vi "LDA_IP.vi"() -> (15 "error out":errorcluster)   [LabVIEW 2013]
uses:
  Globals/Meas_global.vi
  Globals/LDA_meas_global_1.vi
  Globals/LDA_meas_global_2.vi
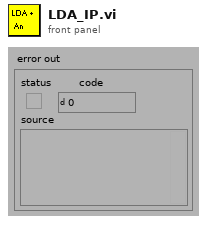
[diagram p1: front panel]
types:
  T1 = typedef "Ch_and_Spans.ctl" = cluster{"high limit (10V)":sgl, "low limit (-10V)":sgl, "Ch No":i16, "Var name":string, "Use Latest Calib":bool}
  T2 = typedef "LDA_Setup.ctl" = cluster{"dimensions":enum16{"1D", "2D"}, "Analogue Freq Multiplier":dbl}
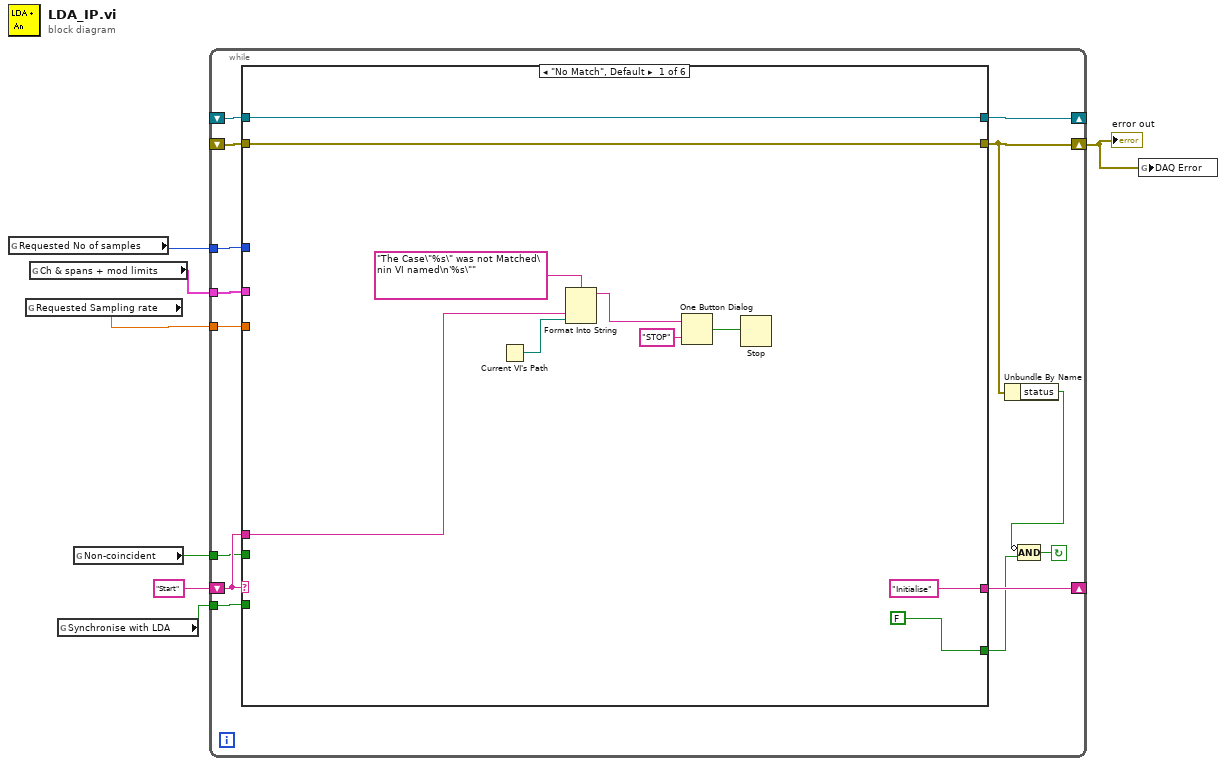
[diagram p0: block diagram]
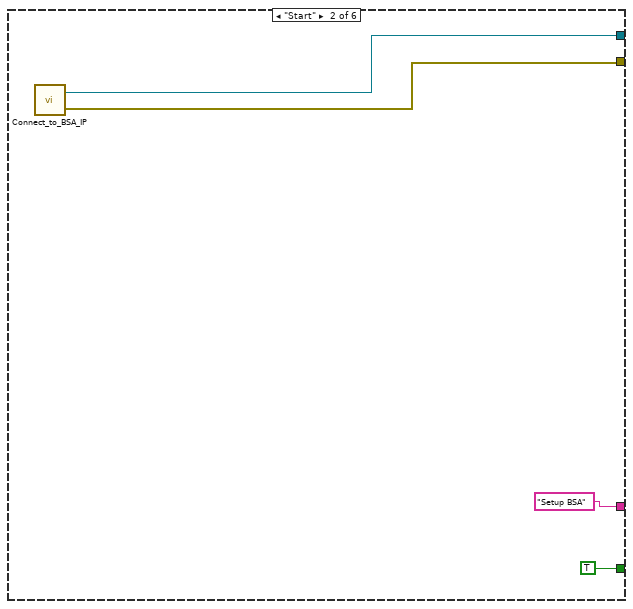
[diagram p2: hidden frame]
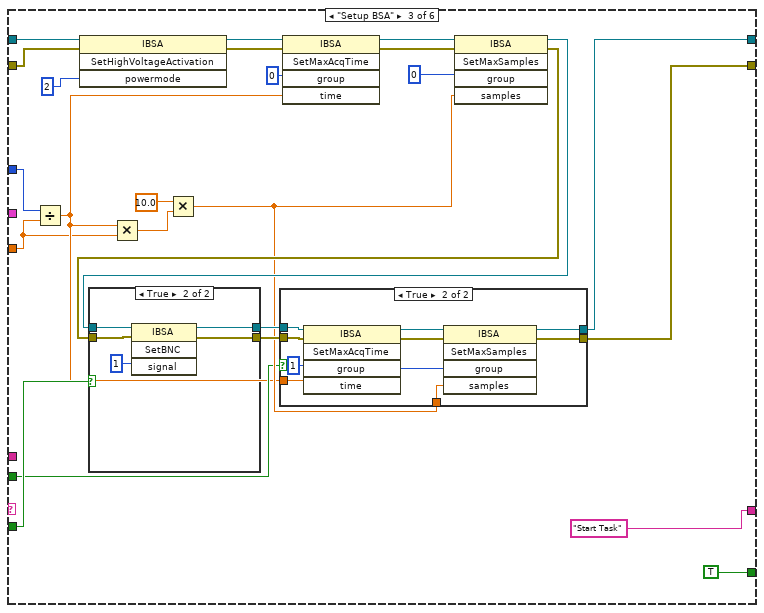
[diagram p3: hidden frame]
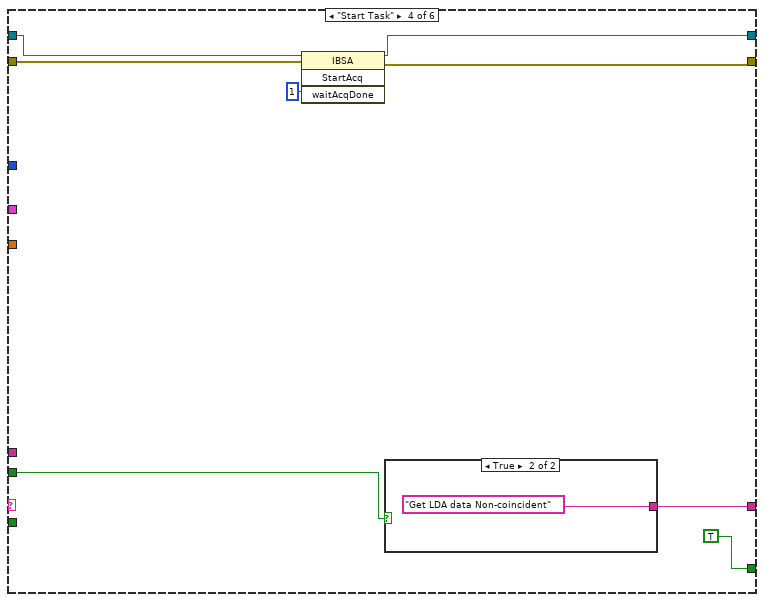
[diagram p6: hidden frame]
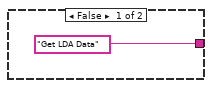
[diagram p7: hidden frame]
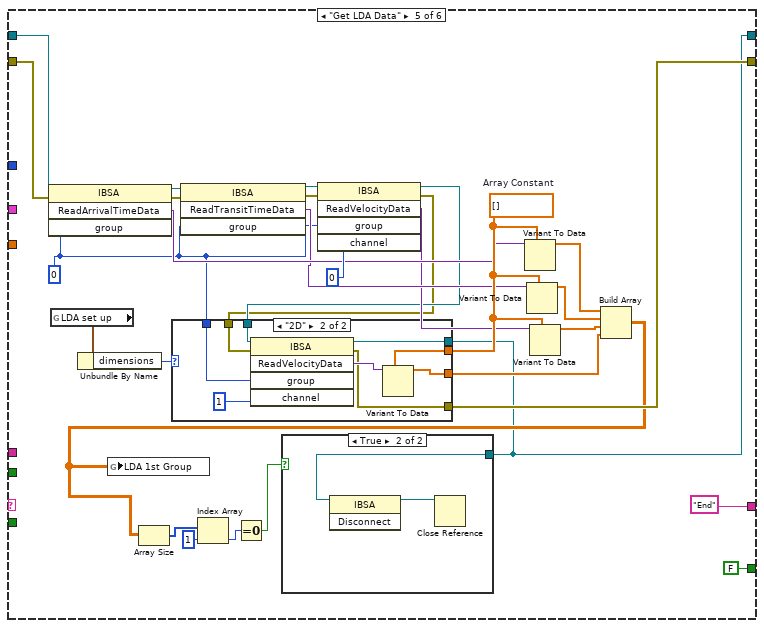
[diagram p8: hidden frame]
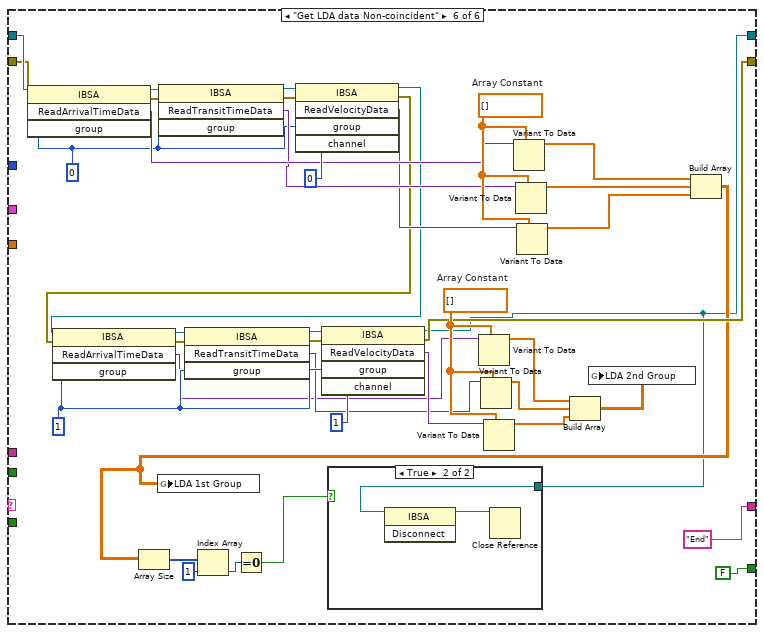
[diagram p11: hidden frame]
diagram:
  n1 = global read "Meas_global.vi" "Requested No of samples"() -> (w2:i32)
  n2 = global read "Meas_global.vi" "Requested Sampling rate"() -> (w3:dbl)
  n3 = global read "Meas_global.vi" "Ch & spans + mod limits"() -> (w4:T1[])
  n4 = global read "Meas_global.vi" "Synchronise with LDA"() -> (w6:bool)
  n5 = global read "LDA_meas_global_1.vi" "Non-coincident"() -> (w5:bool)
  n6 = while {
    shift-left: "Start" -> [w20]
    shift-right: [w21] -> _
    shift-right: [w11] -> w1
    shift-left: _ -> [w19]
    tunnel: w2 -> [w18]
    tunnel: w4 -> [w17]
    tunnel: w3 -> [w16]
    shift-right: [w14] -> _
    shift-left: _ -> [w15]
    tunnel: w6 -> [w13]
    tunnel: w5 -> [w12]
    stop <- w9 continue-if-true
    n7 = case shown="\"No Match\", Default" w20 {
      tunnel: [FALSE TRUE TRUE TRUE FALSE FALSE] -> w8
      tunnel: ["Initialise" "Setup BSA" "Start Task" w81 "End" "End"] -> w21
      tunnel: w20 -> [w26 _ _ _ _ _]
      tunnel: [w23 w33 w42 w85 w100 w142] -> w11
      tunnel: w19 -> [w23 _ w51 w82 w94 w140]
      tunnel: w18 -> [_ _ w52 _ _ _]
      tunnel: w17 -> [_ _ _ _ _ _]
      tunnel: w16 -> [_ _ w37 _ _ _]
      tunnel: w15 -> [w22 _ w53 w84 w104 w141]
      tunnel: [w22 w34 w44 w83 w90 w133] -> w14
      tunnel: w13 -> [_ _ w46 _ _ _]
      tunnel: w12 -> [_ _ w40 w80 _ _]
      frame "No Match", Default {
        n8 = Current VI's Path() -> (path=w25:path)
        n9 = Format Into String(format string="The Case\"%s\" was not Matched\nin VI named\n'%s\"" ("Format String"), w26, w25) -> (resulting string=w29:string)  [unwired: 2 in, 1 out]
        n10 = One Button Dialog(message=w29, button name ("OK")="STOP") -> (true=w27:bool)
        n11 = Stop(stop? (T)=w27) -> ()
      }
      frame "Start" {
        n12 = call "Connect_to_BSA_IP.vi"() -> ("error out"=w33:errorcluster, "BSA"=w34:refnum<k7>)  [unwired: 2 out]
      }
      frame "Setup BSA" {
        n13 = Divide(x=w52, y=w37) -> (x/y=w38:dbl)
        n14 = invoke class="IBSA" method="SetHighVoltageActivation"(reference=w53, error in=w51, "powermode"=2) -> (reference out=w58:refnum<k7>, error out=w60:errorcluster)  [unwired: 1 in, 2 out]
        n15 = Multiply(x=w38, y=w37) -> (x*y=w36:dbl)
        n16 = Multiply(x=10.0 ("y"), y=w36) -> (x*y=w41:dbl)
        n17 = invoke class="IBSA" method="SetMaxAcqTime"(reference=w58, error in=w60, "group"=0, "time"=w38) -> (reference out=w59:refnum<k7>, error out=w57:errorcluster)  [unwired: 1 in, 3 out]
        n18 = invoke class="IBSA" method="SetMaxSamples"(reference=w59, error in=w57, "group"=0, "samples"=w41) -> (reference out=w48:refnum<k7>, error out=w47:errorcluster)  [unwired: 1 in, 3 out]
        n19 = case shown="True" w46 {
          tunnel: w48 -> [w72 w77]
          tunnel: w47 -> [w73 w76]
          tunnel: [w72 w75] -> w45
          tunnel: [w73 w74] -> w43
          frame False {
          }
          frame True {
            n20 = invoke class="IBSA" method="SetBNC"(reference=w77, error in=w76, "signal"=1) -> (reference out=w75:refnum<k7>, error out=w74:errorcluster)  [unwired: 1 in, 2 out]
          }
        }
        n21 = case shown="True" w40 {
          tunnel: w45 -> [w62 w69]
          tunnel: [w62 w67] -> w44
          tunnel: w43 -> [w61 w66]
          tunnel: [w61 w65] -> w42
          tunnel: w38 -> [_ w64]
          tunnel: w41 -> [_ w63]
          frame False {
          }
          frame True {
            w70 = 1 ("group")
            n22 = invoke class="IBSA" method="SetMaxAcqTime"(reference=w69, error in=w66, "group"=w70, "time"=w64) -> (reference out=w68:refnum<k7>, error out=w71:errorcluster)  [unwired: 1 in, 3 out]
            n23 = invoke class="IBSA" method="SetMaxSamples"(reference=w68, error in=w71, "group"=w70, "samples"=w63) -> (reference out=w67:refnum<k7>, error out=w65:errorcluster)  [unwired: 1 in, 3 out]
          }
        }
      }
      frame "Start Task" {
        n24 = invoke class="IBSA" method="StartAcq"(reference=w84, error in=w82, "waitAcqDone"=1) -> (reference out=w83:refnum<k7>, error out=w85:errorcluster)  [unwired: 1 in, 2 out]
        n25 = case shown="True" w80 {
          tunnel: ["Get LDA Data" "Get LDA data Non-coincident"] -> w81
          frame False {
          }
          frame True {
          }
        }
      }
      frame "Get LDA Data" {
        w112 = dbl[] []  # Array Constant
        w101 = 0 ("group")
        n26 = invoke class="IBSA" method="ReadArrivalTimeData"(reference=w104, error in=w94, "group"=w101) -> (reference out=w117:refnum<k7>, error out=w116:errorcluster, "ReadArrivalTimeData"=w111:variant)  [unwired: 1 in, 1 out]
        n27 = global read "Meas_global.vi" "LDA set up"() -> (w93:T2)
        n28 = Unbundle By Name(w93) -> ("dimensions"=w92:enum16{"1D", "2D"})
        n29 = invoke class="IBSA" method="ReadTransitTimeData"(reference=w117, error in=w116, "group"=w101) -> (reference out=w115:refnum<k7>, error out=w114:errorcluster, "ReadTransitTimeData"=w110:variant)  [unwired: 1 in, 1 out]
        n30 = invoke class="IBSA" method="ReadVelocityData"(reference=w115, error in=w114, "group"=w101, "channel"=0) -> (reference out=w103:refnum<k7>, error out=w102:errorcluster, "ReadVelocityData"=w109:variant)  [unwired: 1 in, 2 out]
        n31 = case shown="\"2D\"" w92 {
          tunnel: w112 -> [w121 w130]
          tunnel: [w121 w128] -> w105
          tunnel: [w122 w127] -> w90
          tunnel: w103 -> [w122 w126]
          tunnel: w102 -> [w120 w125]
          tunnel: w101 -> [_ w124]
          tunnel: [w120 w123] -> w100
          frame "1D" {
          }
          frame "2D" {
            n32 = invoke class="IBSA" method="ReadVelocityData"(reference=w126, error in=w125, "group"=w124, "channel"=1) -> (reference out=w127:refnum<k7>, error out=w123:errorcluster, "ReadVelocityData"=w129:variant)  [unwired: 1 in, 2 out]
            n33 = Variant To Data(type=w130, Variant=w129) -> (data=w128:dbl[])  [unwired: 1 in, 1 out]
          }
        }
        n34 = Variant To Data(type=w112, Variant=w111) -> (data=w108:dbl[])  [unwired: 1 in, 1 out]
        n35 = Variant To Data(type=w112, Variant=w110) -> (data=w107:dbl[])  [unwired: 1 in, 1 out]
        n36 = Variant To Data(type=w112, Variant=w109) -> (data=w106:dbl[])  [unwired: 1 in, 1 out]
        n37 = Build Array(w108, w107, w106, w105) -> (w95:dbl[][])
        n38 = global write "LDA_meas_global_2.vi" "LDA 1st Group"(w95) -> ()
        n39 = Array Size(array=w95) -> (size(s)=w99:i32[])
        n40 = Index Array(array=w99, index=1) -> (element=w97:i32)
        n41 = Equal To 0?(x=w97) -> (x = 0?=w96:bool)
        n42 = case shown="True" w96 {
          tunnel: w90 -> [_ w118]
          frame False {
          }
          frame True {
            n43 = invoke class="IBSA" method="Disconnect"(reference=w118) -> (reference out=w119:refnum<k7>)  [unwired: 2 in, 2 out]
            n44 = Close Reference(reference=w119) -> ()  [unwired: 1 in, 1 out]
          }
        }
      }
      frame "Get LDA data Non-coincident" {
        w149 = dbl[] []  # Array Constant
        w156 = 1 ("group")
        w163 = dbl[] []  # Array Constant
        w157 = 0 ("group")
        n45 = invoke class="IBSA" method="ReadArrivalTimeData"(reference=w141, error in=w140, "group"=w157) -> (reference out=w168:refnum<k7>, error out=w167:errorcluster, "ReadArrivalTimeData"=w162:variant)  [unwired: 1 in, 1 out]
        n46 = invoke class="IBSA" method="ReadTransitTimeData"(reference=w168, error in=w167, "group"=w157) -> (reference out=w166:refnum<k7>, error out=w165:errorcluster, "ReadTransitTimeData"=w161:variant)  [unwired: 1 in, 1 out]
        n47 = invoke class="IBSA" method="ReadVelocityData"(reference=w166, error in=w165, "group"=w157, "channel"=0) -> (reference out=w143:refnum<k7>, error out=w144:errorcluster, "ReadVelocityData"=w160:variant)  [unwired: 1 in, 2 out]
        n48 = invoke class="IBSA" method="ReadArrivalTimeData"(reference=w143, error in=w144, "group"=w156) -> (reference out=w151:refnum<k7>, error out=w152:errorcluster, "ReadArrivalTimeData"=w145:variant)  [unwired: 1 in, 1 out]
        n49 = invoke class="IBSA" method="ReadTransitTimeData"(reference=w151, error in=w152, "group"=w156) -> (reference out=w153:refnum<k7>, error out=w154:errorcluster, "ReadTransitTimeData"=w146:variant)  [unwired: 1 in, 1 out]
        n50 = invoke class="IBSA" method="ReadVelocityData"(reference=w153, error in=w154, "group"=w156, "channel"=1) -> (reference out=w133:refnum<k7>, error out=w142:errorcluster, "ReadVelocityData"=w147:variant)  [unwired: 1 in, 2 out]
        n51 = Variant To Data(type=w149, Variant=w145) -> (data=w150:dbl[])  [unwired: 1 in, 1 out]
        n52 = Variant To Data(type=w149, Variant=w146) -> (data=w148:dbl[])  [unwired: 1 in, 1 out]
        n53 = Variant To Data(type=w149, Variant=w147) -> (data=w137:dbl[])  [unwired: 1 in, 1 out]
        n54 = Variant To Data(type=w163, Variant=w162) -> (data=w159:dbl[])  [unwired: 1 in, 1 out]
        n55 = Variant To Data(type=w163, Variant=w161) -> (data=w158:dbl[])  [unwired: 1 in, 1 out]
        n56 = Variant To Data(type=w163, Variant=w160) -> (data=w138:dbl[])  [unwired: 1 in, 1 out]
        n57 = Build Array(w150, w148, w137) -> (w139:dbl[][])
        n58 = global write "LDA_meas_global_2.vi" "LDA 2nd Group"(w139) -> ()
        n59 = Build Array(w159, w158, w138) -> (w136:dbl[][])
        n60 = Array Size(array=w136) -> (size(s)=w171:i32[])
        n61 = global write "LDA_meas_global_2.vi" "LDA 1st Group"(w136) -> ()
        n62 = Index Array(array=w171, index=1) -> (element=w169:i32)
        n63 = Equal To 0?(x=w169) -> (x = 0?=w135:bool)
        n64 = case shown="True" w135 {
          tunnel: w133 -> [_ w173]
          frame False {
          }
          frame True {
            n65 = invoke class="IBSA" method="Disconnect"(reference=w173) -> (reference out=w172:refnum<k7>)  [unwired: 2 in, 2 out]
            n66 = Close Reference(reference=w172) -> ()  [unwired: 1 in, 1 out]
          }
        }
      }
    }
    n67 = Unbundle By Name(w11) -> ("status"=w10:bool)
    n68 = Compound Arithmetic op=AND(invert w10, w8) -> (w9:bool)
  }
  "error out" <- w1
  n69 = global write "Meas_global.vi" "DAQ Error"(w1) -> ()
